vi "Set Active Chassis.vi"(8 "error in (no error)":errorcluster, 9 "Rfrsh GUI? (T)":bool=TRUE, 10 "Chassis Name":string, 11 "Cfg Grandmaster in":refnum<class "Cfg Grandmaster.lvclass">) -> (0 "error out":errorcluster, 3 "Cfg Grandmaster out":refnum<class "Cfg Grandmaster.lvclass">)   [LabVIEW 2018, in "Configuration Grandmaster.lvlib" / "Cfg Grandmaster.lvclass"]
uses:
  Cfg Grandmaster.lvclass
  Cfg Grandmaster.lvclass/Cfg Grandmaster.ctl
  Class Chassis BOM/Chassis BOM.lvclass/Chassis BOM.ctl
  Class Chassis BOM/Read Chassis Alias.vi
  Class Chassis BOM/Chassis BOM.lvclass
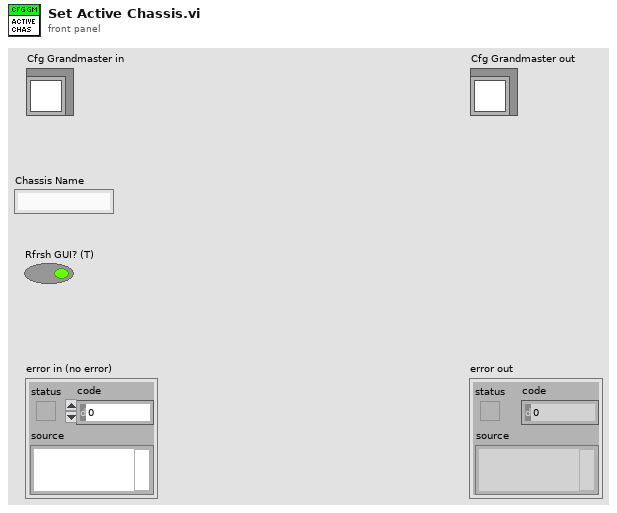
[diagram p1: front panel]
types:
  T1 = typedef "ge_Cfg wChassis.ctl" = cluster{"Chassis BOM":refnum<class "Chassis BOM.lvclass">, "Chassis Cfg":refnum<class "ChassisCfg.lvclass">, "Chassis Tasks":refnum<class "Chassis Tasks.lvclass">, "HW Error":bool, "Unsvd Chgs?":bool}
  T2 = typedef "Selected Group.ctl" = cluster{"ChanGroup":i32, "Rate Class":T3}
  T3 = typedef "TE_Designator.ctl" = enum16{"High Speed", "Low Speed"}
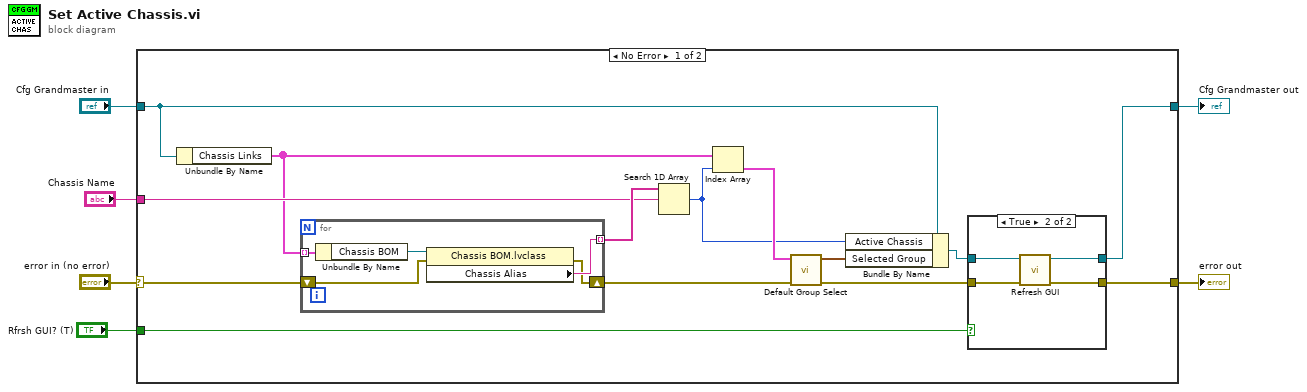
[diagram p0: block diagram]
diagram:
  n1 = case shown="No Error" "error in (no error)" {
    selector: "error in (no error)" -> [w18 w33]
    tunnel: [w10 w33] -> w5
    tunnel: [w9 w32] -> w3
    tunnel: "Cfg Grandmaster in" -> [w14 w32]
    tunnel: "Chassis Name" -> [w19 _]
    tunnel: "Rfrsh GUI? (T)" -> [w8 _]
    frame No Error {
      n2 = Unbundle By Name(w14) -> ("Chassis Links"=w17:T1[])
      n3 = for {
        tunnel: w17 -> [w31] mode=indexing
        tunnel: [w29] -> w20 mode=indexing
        shift-right: [w27] -> w16
        shift-left: w18 -> [w28]
        n4 = Unbundle By Name(w31) -> ("Chassis BOM"=w30:refnum<class "Chassis BOM.lvclass">)
        n5 = property class="Chassis BOM.lvclass"(reference=w30, error in=w28) -> (error out=w27:errorcluster, "Chassis Alias"=w29:string)  [unwired: 1 out]
      }
      n6 = Search 1D Array(1D array=w20, element=w19) -> (index of element=w7:i32)  [unwired: 1 in]
      n7 = Index Array(array=w17, index=w7) -> (element=w15:T1)
      n8 = call "Default Group Select.vi"("error in"=w16, "Cfg with Chassis"=w15) -> ("error out"=w12:errorcluster, "Selected Grp"=w13:T2)  [unwired: 8 in]
      n9 = Bundle By Name(cluster=w14, "Active Chassis"=w7, "Selected Group"=w13) -> (w11:refnum<class "Cfg Grandmaster.lvclass">)
      n10 = case shown="True" w8 {
        tunnel: w12 -> [w21 w26]
        tunnel: w11 -> [w22 w25]
        tunnel: [w21 w23] -> w10
        tunnel: [w22 w24] -> w9
        frame False {
        }
        frame True {
          n11 = call "Refresh GUI.vi"("error in (no error)"=w26, "Cfg Grandmaster in"=w25) -> ("error out"=w23:errorcluster, "Cfg Grandmaster out"=w24:refnum<class "Cfg Grandmaster.lvclass">)  [unwired: 8 in]
        }
      }
    }
    frame Error {
    }
  }
  "error out" <- w5
  "Cfg Grandmaster out" <- w3
